vi "getWavelength.vi"(8 "error in (no error)":errorcluster, 9 "Monochromator in":refnum<class "Monochromator.lvclass">, 11 "MonoState in":refnum<class "MonoState.lvclass">) -> (0 "error out":errorcluster, 1 "Monochromator out":refnum<class "Monochromator.lvclass">, 2 "wavelength":T1, 3 "MonoState out":refnum<class "MonoState.lvclass">)   [LabVIEW 2020, in "MonoState.lvclass"]
uses:
  MonoState.lvclass
  Typedefs/wavelength.ctl
  Monochromator/Monochromator.lvclass
  Monochromator/Monochromator.lvclass/Monochromator.ctl
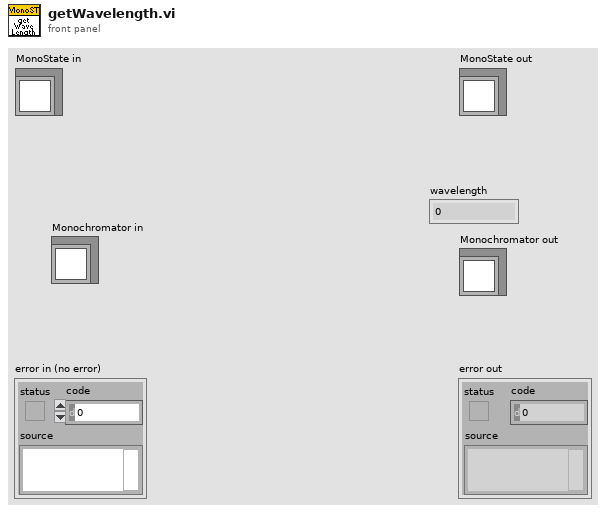
[diagram p1: front panel]
types:
  T1 = typedef "wavelength.ctl" = dbl
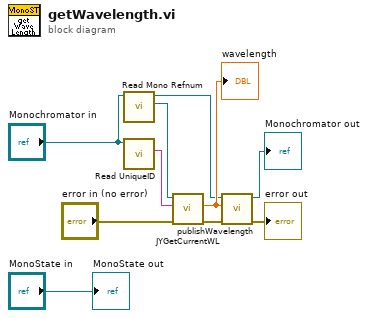
[diagram p0: block diagram]
diagram:
  n1 = call "Read Mono Refnum.vi"("Monochromator in"="Monochromator in") -> ("Mono Refnum"=w3:refnum<k7>, "Monochromator out"=w2:refnum<class "Monochromator.lvclass">)  [unwired: 8 in, 1 out]
  n2 = call "Read UniqueID.vi"("Monochromator in"="Monochromator in") -> ("UniqueID"=w1:string)  [unwired: 8 in, 2 out]
  n3 = call "JYGetCurrentWL.vi"("error in (no error)"="error in (no error)", "UniqueID"=w1, "JYMONOLib.IJYMonoReqd"=w3) -> ("error out"=w4:errorcluster, "Current WL"=w5:dbl)  [unwired: 5 in, 2 out]
  "wavelength" <- w5
  n4 = call "publishWavelength.vi"("error in (no error)"=w4, "wavelength"=w5, "Monochromator in"=w2) -> ("error out"=→"error out":errorcluster, "Monochromator out"=→"Monochromator out":refnum<class "Monochromator.lvclass">)  [unwired: 7 in]
  "MonoState out" <- "MonoState in"
